vi "initialise_old.vi"(8 "error in (no error)":errorcluster, 11 "DL090211ImageAssemblerScaffold in":refnum<class "ImageAssemblerDL090211Scaffold.lvclass">) -> (0 "error out":errorcluster, 3 "DL090211ImageAssemblerScaffold out":refnum<class "ImageAssemblerDL090211Scaffold.lvclass">)   [LabVIEW 2010]
doc: "The dynamic dispatch-version of this VI initalises the plug-in object by allocating and initalising any dynamic resources need."
uses:
  common/classes/Image/Image/Image.lvclass
  ImageAssemblerDL090211Scaffold.lvclass
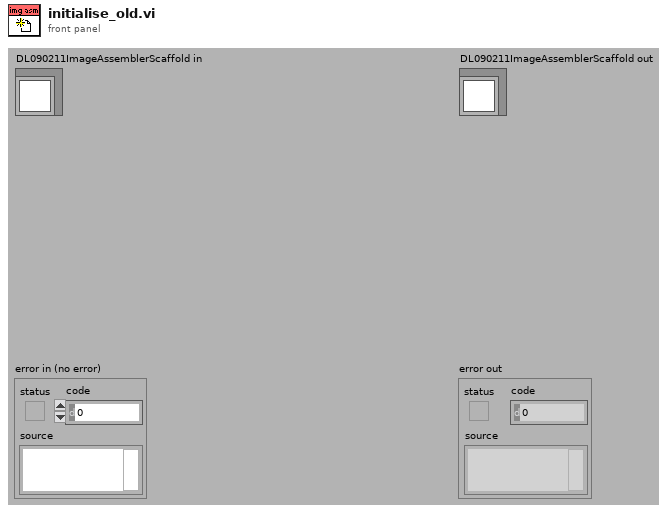
[diagram p1: front panel]
types:
  T1 = typedef "Image Type" = u32
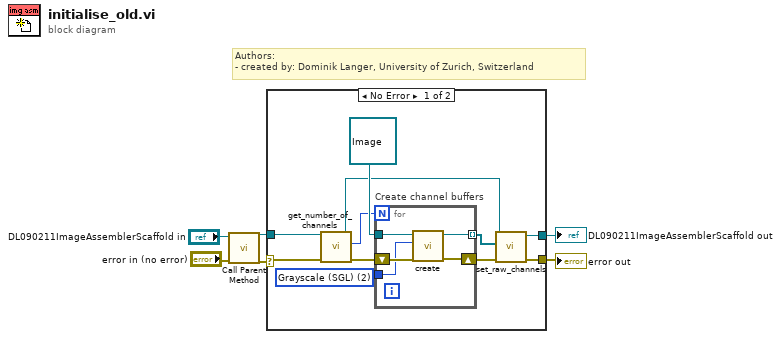
[diagram p0: block diagram]
diagram:
  # "Authors: \n- created by: Dominik Langer, University of Zurich, Switzerland"
  n1 = call-parent "Call Parent Method"("error in (no error)"="error in (no error)", "GenericPlugin in"="DL090211ImageAssemblerScaffold in") -> ("error out"=w4:errorcluster, "GenericPlugin out"=w1:refnum<class "ImageAssemblerDL090211Scaffold.lvclass">)  [unwired: 8 out]
  n2 = case shown="No Error" w4 {
    selector: w4 -> [w11 w23]
    tunnel: w1 -> [w9 w24]
    tunnel: [w12 w23] -> w6
    tunnel: [w13 w24] -> w5
    frame No Error {
      w14 = T1 2 items=["Grayscale (U8)", "Grayscale (I16)", "Grayscale (SGL)", "Complex (CSG)", "RGB (U32)", "HSL (U32)", "RGB (U64)", "Grayscale (U16)"] ("Image Type")
      n3 = call-dynamic "get_number_of_channels.vi"("error in (no error)"=w11, "GenericImageAssembler.lvclass in"=w9) -> ("error out"=w10:errorcluster, "number of channels"=w7:i32, "GenericImageAssembler.lvclass out"=w8:refnum<class "ImageAssemblerDL090211Scaffold.lvclass">)  [unwired: 7 out]
      n4 = for "Create channel buffers" {
        N: w7 -> [_]
        shift-right: [w20] -> w16
        shift-left: w10 -> [w22]
        tunnel: refnum<class "Image.lvclass"> refnum ("Image.lvclass") -> [w21]
        tunnel: [w19] -> w15 mode=indexing
        tunnel: w14 -> [w18]
        n5 = call "create.vi"("error in (no error)"=w22, "Image Type"=w18, "Image in"=w21) -> ("error out"=w20:errorcluster, "Image out"=w19:refnum<class "Image.lvclass">)  [unwired: 1 in, 6 out]
      }
      n6 = call "set_raw_channels.vi"("error in (no error)"=w16, "raw channels"=w15, "DL090211ImageAssemblerScaffold.lvclass in"=w8) -> ("error out"=w12:errorcluster, "DL090211ImageAssemblerScaffold.lvclass out"=w13:refnum<class "ImageAssemblerDL090211Scaffold.lvclass">)  [unwired: 7 out]
    }
    frame Error {
    }
  }
  "error out" <- w6
  "DL090211ImageAssemblerScaffold out" <- w5
